vi "SetAverages_SubVI.vi"(9 "Averages":i32, 10 "instrument handle":refnum<k15>, 11 "VISA Refnum in":refnum<visa-resource-name>) -> (0 "error out":errorcluster)   [LabVIEW 2023, in "SpectrumAnalyzerUI.lvlib" / "SpectrumAnalyzerUI.lvclass"]
uses:
  UIs/SpectrumAnalyzerUI/SpectrumAnalyzerUI/SpectrumAnalyzerUI.lvclass
  UIs/SpectrumAnalyzerUI/SpectrumAnalyzerUI/SpectrumAnalyzerUI.lvclass/SpectrumAnalyzerUI.ctl
  <instrlib>/Keysight XSAn/Keysight XSAn.lvlib
  KeysightN9020B.lvlib
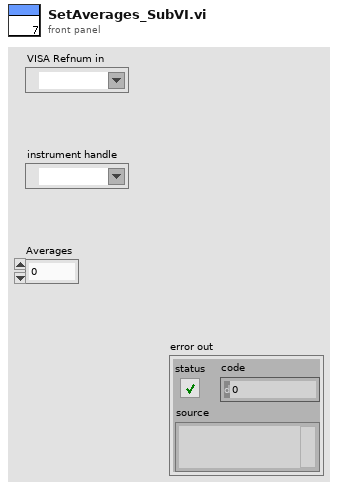
[diagram p1: front panel]
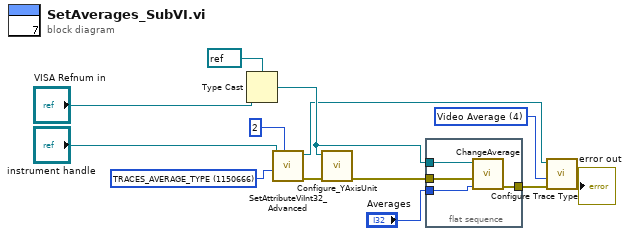
[diagram p0: block diagram]
diagram:
  w4 = u32 1150666 items=["IVILXISYNC_ARM_ALARM_REPEAT_COUNT"=1950004, "IVILXISYNC_ARM_COUNT"=1950007, "IVILXISYNC_ARM_SOURCE_DETECTION"=1950010, "IVILXISYNC_EVENT_DRIVE_MODE"=1950030, "IVILXISYNC_EVENT_SLOPE"=1950031, "IVILXISYNC_EVENT_WIRED_OR_BIAS_MODE"=1950033, "IVILXISYNC_TRIGGER_ALARM_REPEAT_COUNT"=1950018, "IVILXISYNC_TRIGGER_COUNT"=1950021, "IVILXISYNC_TRIGGER_SOURCE_DETECTION"=1950025, "LEVEL_ATTENUATION_OPTIMIZE"=1150012, "LEVEL_ATTENUATION_STEP_INCREMENT"=1150013, "LEVEL_ELECTRONIC_ATTENUATION"=1150578, "MEMORYOPERATION_SCREEN_IMAGE_THEME"=1150678, "NUMBER_OF_SWEEPS"=1250010, "OUTPUT_ANALOG_TYPE"=1150679, "OUTPUT_AUXILIARY_IF_TYPE"=1150681, "PRESELECTOR_MW_PATH"=1150585, "RADIO_BAND_CLASS"=1150550, "RADIO_DEVICE"=1150547, "RADIO_NON_STANDARD_MEASUREMENT_ENABLED"=1150549, "RADIO_PACKET_TYPE"=1150551, "RADIO_STANDARD"=1150548, "REFOSCILLATOR_EXTERNAL_BANDWIDTH"=1150539, "REFOSCILLATOR_EXTERNAL_COUPLING"=1150538, "REFOSCILLATOR_SOURCE "=1150877, "STATETRIGGER_DETECTION"=1150159, "SYSTEM_IO_TIMEOUT"=1150783, "SYSTEM_TIMEOUT_MILLISECONDS"=1150175, "TRACE_DETECTOR_TYPE"=1150782, "TRACE_TYPE"=1250020, "TRACES_AVERAGE_TYPE"=1150666, "TRIGGER_EXTERNAL2_SLOPE"=1150671, "TRIGGER_EXTERNAL_SLOPE"=1150803, "TRIGGER_FRAME_SYNC_SOURCE"=1150841, "TRIGGER_LINE_DELAY_SLOPE"=1150836, "TRIGGER_RFBURST_SLOPE "=1150830, "TRIGGER_SOURCE"=1250301, "TRIGGER_VIDEO_SLOPE"=1150806, "VERTICAL_SCALE"=1250021, "VIDEO_TRIGGER_SLOPE"=1250502] ("AttributeID")
  w9 = 4 items=["Clear Write"=1, "Maximum Hold"=2, "Minimum Hold"=3, "Video Average"=4, "View"=5, "Store"=6] ("trace type (Clear Write)")
  n1 = Type Cast(type=refnum<visa-resource-name> refnum ("VISA resource name"), x="VISA Refnum in") -> (*(type *) &x=w12:refnum<visa-resource-name>)
  n2 = call <instrlib>:"SetAttributeViInt32_Advanced.vi"("AttributeValue"=2, "AttributeID"=w4, "instrument handle"="instrument handle") -> ("error out"=w2:errorcluster, "instrument handle out"=w10:refnum<k15>)  [unwired: 7 in]
  n3 = call "Configure_YAxisUnit.vi"("error in (no error)"=w2, "VISA resource name"=w12) -> ("error out"=w6:errorcluster)  [unwired: 9 in]
  n4 = flat-sequence {
    tunnel: w6 -> [w17]
    tunnel: [w16] -> w1
    tunnel: "Averages" -> [w15]
    tunnel: w12 -> [w14]
    frame #0 {
      n5 = call "ChangeAverage.vi"("Averages"=w15, "error in (no error)"=w17, "VISA resource name"=w14) -> ("error out"=w16:errorcluster)  [unwired: 8 in]
    }
  }
  n6 = call <instrlib>:"Configure Trace Type.vi"("error in (no error)"=w1, "trace type (Clear Write)"=w9, "instrument handle"=w10) -> ("error out"=→"error out":errorcluster)  [unwired: 7 in, 1 out]
